vi "Read configuration.vi"(8 "error in (no error)":errorcluster, 11 "ACIR Channel":refnum<class "SwitchACIR Channel.lvclass">) -> (0 "error out":errorcluster, 2 "configuration":refnum<class "CEF_serializable configuration.lvclass">, 3 "ACIR Channel out":refnum<class "SwitchACIR Channel.lvclass">)   [LabVIEW 2025, in "SwitchACIR Channel.lvclass"]
uses:
  SwitchACIR Channel.lvclass
  Users/Public/Documents/Sandia National Labs/TSS Plugin/CEF.lvlibp/serializable configuration/CEF_serializable configuration.lvclass
  SwitchACIR Channel.lvclass/SwitchACIR Channel.ctl
  SwitchACIR Channel configuration/SwitchACIR Channel configuration.lvclass
  C:/Users/Public/Documents/Sandia National Labs/TSS Plugin/CEF.lvlibp/serializable configuration/CEF_serializable configuration.lvclass
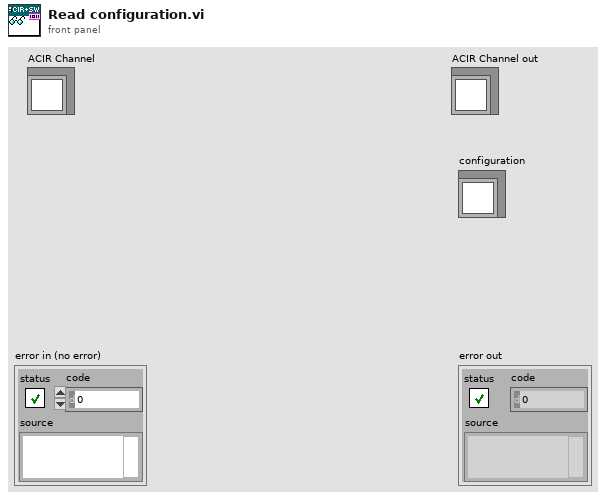
[diagram p1: front panel]
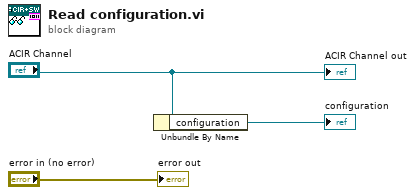
[diagram p0: block diagram]
diagram:
  n1 = Unbundle By Name("ACIR Channel") -> ("configuration"=→"configuration":refnum<class "SwitchACIR Channel configuration.lvclass">)
  "error out" <- "error in (no error)"
  "ACIR Channel out" <- "ACIR Channel"
